vi "9871 EPICS Test 20220801.vi"() -> ()   [LabVIEW 2021]
doc: "This is the top level VI for a cRIO target. This example will perform a read and a write from the same port on the 987x module. You can use this VI to verify that the port is working correctly. It uses two DMA channels for communication, one channel from the FPGA to the controller and one channel from the controller to the FPGA. For this reason a cRIO-900x contoller can not be used with this VI. You must use the other examples in this program as they only use DMA from the FPGA to the controller, which is supported by all cRIO controllers.\n\nPlease see the block diagram for more detailed comments."
uses:
  <vilib>/LabVIEW Targets/FPGA/cRIO/shared/nicrio_ModuleControls/nicrio_cRIO-9871_BaudRateEnum.ctl
  <vilib>/LabVIEW Targets/FPGA/cRIO/shared/nicrio_ModuleControls/nicrio_cRIO-9871_DataBitsEnum.ctl
  <vilib>/LabVIEW Targets/FPGA/cRIO/shared/nicrio_ModuleControls/nicrio_cRIO-9871_FlowControlEnum.ctl
  <vilib>/LabVIEW Targets/FPGA/cRIO/shared/nicrio_ModuleControls/nicrio_cRIO-9871_ParityEnum.ctl
  <vilib>/LabVIEW Targets/FPGA/cRIO/shared/nicrio_ModuleControls/nicrio_cRIO-9871_StopBitsEnum.ctl
  <vilib>/FPGAPlugInAG/cRIO-9048/niLvFpga_Open_cRIO-9048.vi
  <vilib>/FPGAPlugInAG/cRIO-9048/niLvFpga_Reset_cRIO-9048.vi
  <vilib>/FPGAPlugInAG/cRIO-9048/niLvFpga_Run_cRIO-9048.vi
  <vilib>/Utility/error.llb/Error Cluster From Error Code.vi
  <vilib>/rvi/errors/niLvFpgaAdjustHostInterfaceError.vi
  <vilib>/FPGAPlugInAG/cRIO-9048/niLvFpga_Close_cRIO-9048.vi
  <vilib>/rvi/interface/nirviOpenFPGA/nirviOpenFPGA.xnode
  FPGA Bitfiles/testFIFO_20220801.lvbitx
  <vilib>/rvi/interface/nirviMethod/nirviMethod.xnode
  <vilib>/rvi/interface/nirviReadWriteControl/nirviReadWriteControl.xnode
  <vilib>/rvi/interface/nirviCloseFPGA/nirviCloseFPGA.xnode
  <vilib>/rvi/errors/niLvFpgaMergeErrorWithErrorCode.vi
  <vilib>/FPGAPlugInAG/cRIO-9048/niLvFpga_WriteFifo_cRIO-9048.vi
  NiFpgaLv.dll
panel:
  out "index":fxp<+,4,4>
  out "Array":u16[](array[numeric])
  out "LoopCount":i32
  out "FIFO Timeout 2MTicks=50ms":i32
  out "Port Bits Only in U16":u16
  out "Port# (1-4) 2":u8
  out "Parameter High Nibble Mid 4 bits  (xxNNNNxx xxxxxxxx)":u8
  out "Low Byte (xxxxxxxx NNNNNNNN)":u8
  out "Element":u16
  out "error out":errorcluster
  in  "reset":bool
  in  "error in":errorcluster
  in  "Stop Bits":T1
  in  "Parity":T2
  in  "Flow Control":T3
  in  "Data Bits":T4=enum."8"
  in  "Baud Rate":T5=enum."9600 bps" caption="Baud"
  in  "Port# (1-4)":u8=1 min=1 max=4
  in  "Request Type":T6(ring)
  in  "stop":bool
  in  "Write":bool
  out "WriteError":errorcluster
  out "WrBytesLeft":u32
  in  "Send String":string="ABCDEFGHIJKLMNOPQRSTUVWXYZ-abcdefghijklmnopqrstuvwxyz-0123456789"
  # "Transmit"
  # "Receive"
  # "Parameters"
  # "Write"
  # "Read"
  # "READ"
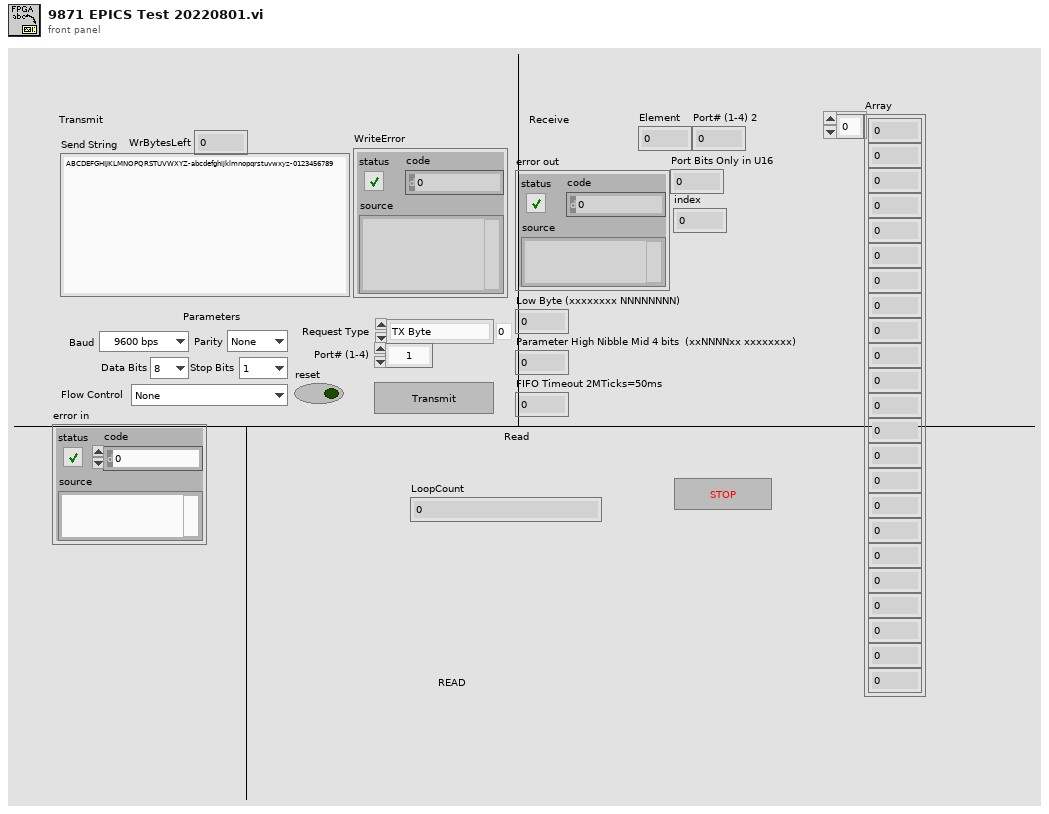
[diagram p1: front panel]
types:
  T1 = typedef "nicrio_cRIO-9871_StopBitsEnum.ctl" = enum8{"1", "1.5", "2"}
  T2 = typedef "nicrio_cRIO-9871_ParityEnum.ctl" = enum8{"None", "Odd", "Even", "Mark", "Space"}
  T3 = typedef "nicrio_cRIO-9871_FlowControlEnum.ctl" = enum8{"None", "Software (XON / XOFF)", "Hardware (RTS / CTS)"}
  T4 = typedef "nicrio_cRIO-9871_DataBitsEnum.ctl" = enum8{"5", "6", "7", "8"}
  T5 = typedef "nicrio_cRIO-9871_BaudRateEnum.ctl" = enum16{"75 bps", "110 bps", "134 bps", "150 bps", "300 bps", "600 bps", "1200 bps", "1800 bps", "2400 bps", "4800 bps", "7200 bps", "9600 bps", "14.4 kbps", "19.2 kbps", "28.8 kbps", "38.4 kbps", "57.6 kbps", "115.2 kbps", "230.4 kbps", "460.8 kbps", "921.6 kbps"}
  T6 = enum16{"TX Byte", "TX Clear", "Echo Request", "Parameter Change"}
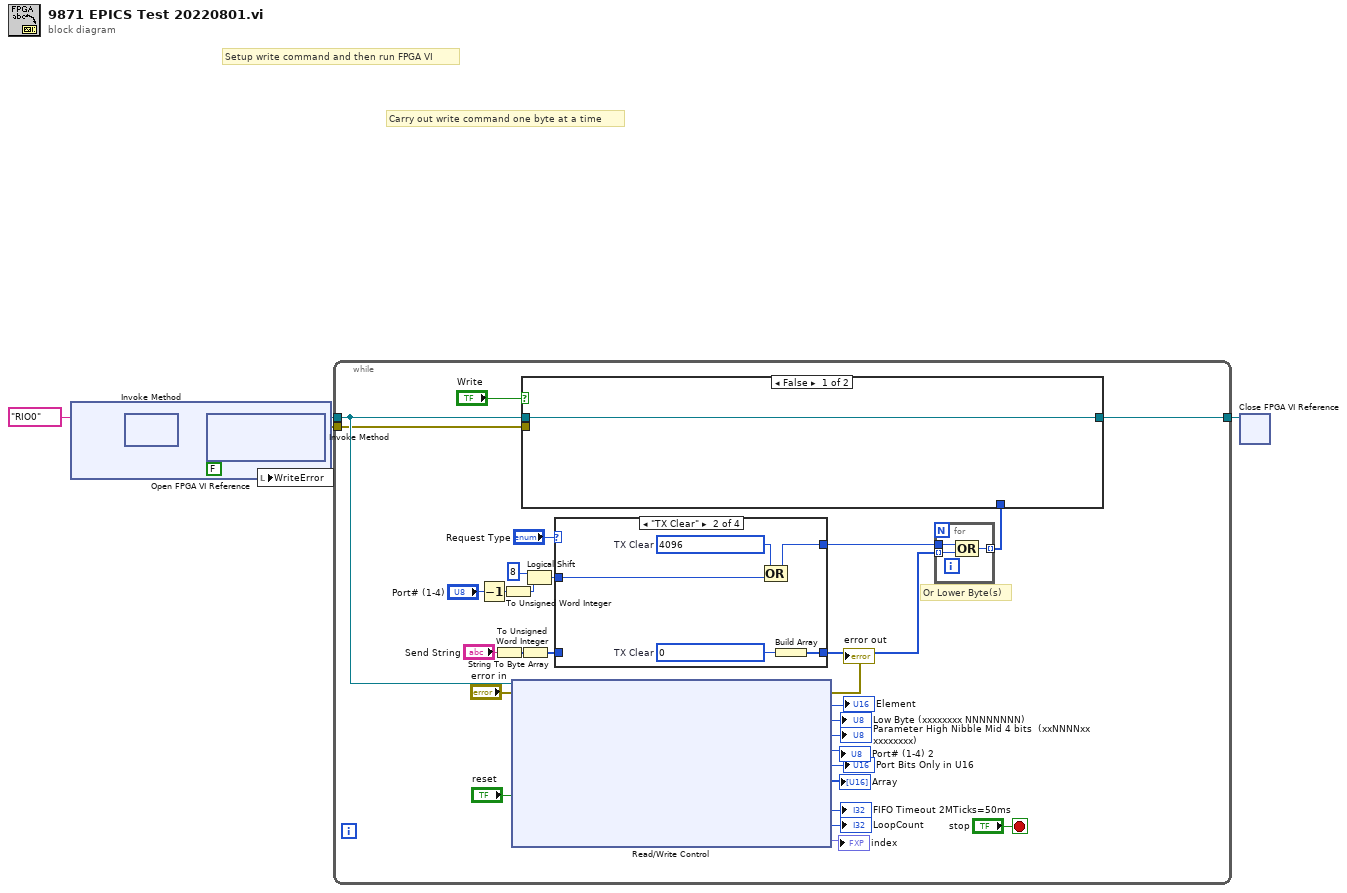
[diagram p0: block diagram]
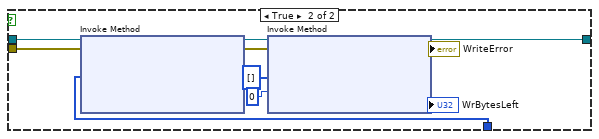
[diagram p2: hidden frame]
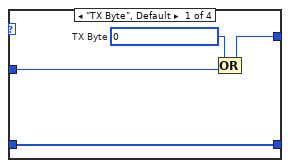
[diagram p3: hidden frame]
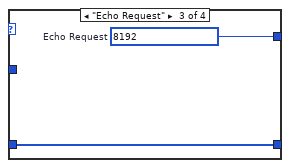
[diagram p4: hidden frame]
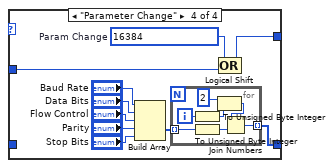
[diagram p5: hidden frame]
diagram:
  # "Carry out write command one byte at a time"
  # "Setup write command and then run FPGA VI"
  n1 = xnode "Open FPGA VI Reference"("resource name"=tag "RIO0") -> ("FPGA VI Reference Out"=w5:refnum<k20>, "error out"=w9:errorcluster)  [unwired: 1 in]
  n2 = xnode "Invoke Method"("FPGA VI Reference In"=w5, "error in"=w9) -> ("FPGA VI Reference Out"=w6:refnum<k20>, "error out"=w7:errorcluster)
  n3 = xnode "Invoke Method"("FPGA VI Reference In"=w6, "error in"=w7, "Wait Until Done (F)"=FALSE) -> ("FPGA VI Reference Out"=w3:refnum<k20>, "error out"=w4:errorcluster)
  n4 = local write "WriteError"(w4) -> ()
  n5 = while {
    tunnel: w4 -> [w23]
    tunnel: w3 -> [w37]
    tunnel: [w36] -> w2
    stop <- "stop" stop-if-true
    # "Or Lower Byte(s)"
    n6 = Decrement(x="Port# (1-4)") -> (x-1=w29:u8)
    n7 = String To Byte Array(string="Send String") -> (unsigned byte array=w25:u8[])
    n8 = To Unsigned Word Integer(number=w29) -> (unsigned 16bit integer=w31:u16)
    n9 = xnode "Read/Write Control"("FPGA VI Reference In"=w37, "error in"="error in", "reset"="reset") -> ("error out"=→"error out":errorcluster, "Element"=→"Element":u16, "Low Byte (xxxxxxxx NNNNNNNN)"=→"Low Byte (xxxxxxxx NNNNNNNN)":u8, "Parameter High Nibble Mid 4 bits  (xxNNNNxx xxxxxxxx)"=→"Parameter High Nibble Mid 4 bits  (xxNNNNxx xxxxxxxx)":u8, "Port# (1-4)"=→"Port# (1-4) 2":u8, "Port Bits Only in U16"=→"Port Bits Only in U16":u16, "Array"=→"Array":u16[], "FIFO Timeout 2MTicks=50ms"=→"FIFO Timeout 2MTicks=50ms":i32, "LoopCount"=→"LoopCount":i32, "index"=→"index":fxp<+,4,4>)  [unwired: 1 out]
    n10 = To Unsigned Word Integer(number=w25) -> (unsigned 16bit integer=w24:u16[])
    n11 = Logical Shift(y=i16 8, x=w31) -> (x << y=w27:u16)
    n12 = case shown="\"TX Clear\"" "Request Type" {
      tunnel: [w52 w56 w60 w63] -> w32
      tunnel: w27 -> [w51 w58 _ w65]
      tunnel: [w50 w55 w59 w61] -> w26
      tunnel: w24 -> [w50 _ w59 _]
      frame "TX Byte", Default {
        w53 = u16 0  # TX Byte
        n13 = Compound Arithmetic op=OR(w53, w51) -> (w52:u16)
      }
      frame "TX Clear" {
        w54 = u16 0  # TX Clear
        w57 = u16 4096  # TX Clear
        n14 = Compound Arithmetic op=OR(w57, w58) -> (w56:u16)
        n15 = Build Array(w54) -> (w55:u16[])
      }
      frame "Echo Request" {
        w60 = u16 8192  # Echo Request
      }
      frame "Parameter Change" {
        w64 = u16 16384  # Param Change
        n16 = Build Array("Baud Rate", "Data Bits", "Flow Control", "Parity", "Stop Bits") -> (w62:u16[])
        n17 = for {
          tunnel: w62 -> [w77] mode=indexing
          tunnel: [w74] -> w61 mode=indexing
          i -> [w75]
          n18 = To Unsigned Byte Integer(number=w75) -> (unsigned 8bit integer=w71:u8)
          n19 = To Unsigned Byte Integer(number=w77) -> (unsigned 8bit integer=w76:u8)
          n20 = Logical Shift(y=i16 2, x=w71) -> (x << y=w72:u8)
          n21 = Join Numbers(hi=w72, lo=w76) -> ((hi.lo)=w74:u16)
        }
        n22 = Compound Arithmetic op=OR(w64, w65) -> (w63:u16)
      }
    }
    n23 = for {
      tunnel: w26 -> [w78] mode=indexing
      tunnel: [w80] -> w35 mode=indexing
      tunnel: w32 -> [w79]
      n24 = Compound Arithmetic op=OR(w79, w78) -> (w80:u16)
    }
    n25 = case shown="False" "Write" {
      tunnel: w37 -> [w39 w49]
      tunnel: [w39 w48] -> w36
      tunnel: w35 -> [_ w41]
      tunnel: w23 -> [_ w40]
      frame False {
      }
      frame True {
        n26 = xnode "Invoke Method"("FPGA VI Reference In"=w49, "error in"=w40, "Data"=w41) -> ("FPGA VI Reference Out"=w45:refnum<k20>, "error out"=w44:errorcluster)  [unwired: 1 in, 1 out]
        n27 = xnode "Invoke Method"("FPGA VI Reference In"=w45, "error in"=w44, "Data"=u16[] [], "Timeout (ms)"=0) -> ("FPGA VI Reference Out"=w48:refnum<k20>, "error out"=→"WriteError":errorcluster, "Empty Elements Remaining"=→"WrBytesLeft":u32)
      }
    }
  }
  n28 = xnode "Close FPGA VI Reference"("FPGA VI Reference In"=w2) -> ()  [unwired: 1 in, 1 out]
